vi "Pre Launch Init.vi"(11 "Series Actor in":refnum<class "Series Actor.lvclass">) -> (0 "error out":errorcluster, 3 "Series Actor out":refnum<class "Series Actor.lvclass">)   [LabVIEW 2023, in "HAL GOOP4.lvlib" / "Series Actor.lvlib" / "Series Actor.lvclass"]
doc: "(<B>Filename</B>: Actor Framework.lvlib:Actor.lvclass:Pre Launch Init.vi)\n\nDefines behavior that occurs after the Launch Nested Actor method is invoked but before the actor's Actor Core method begins running.\n\nBy default, this method does nothing. A descendant class may override it to define behavior."
uses:
  Series Actor.lvclass
  Series Actor.lvclass/Series Actor.ctl
  <vilib>/ActorFramework/Actor/Actor.lvclass
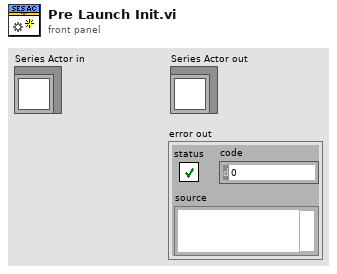
[diagram p1: front panel]
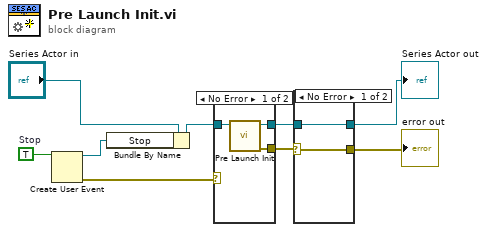
[diagram p0: block diagram]
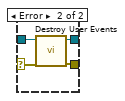
[diagram p2: hidden frame]
diagram:
  w8 = TRUE  # Stop
  n1 = Create User Event(user event datatype=w8) -> (user event=w1:refnum<user-event>, error out=w7:errorcluster)  [unwired: 1 in]
  n2 = Bundle By Name(cluster="Series Actor in", "Stop"=w1) -> (w2:refnum<class "Series Actor.lvclass">)
  n3 = case shown="No Error" w7 {
    selector: w7 -> [_ w14]
    tunnel: [w12 w14] -> w6
    tunnel: [w11 w13] -> w4
    tunnel: w2 -> [w10 w13]
    frame No Error {
      n4 = call-parent "Pre Launch Init.vi"("Actor in"=w10) -> ("error out"=w12:errorcluster, "Actor out"=w11:refnum<class "Series Actor.lvclass">)  [unwired: 9 in]
    }
    frame Error {
    }
  }
  n5 = case shown="No Error" w6 {
    selector: w6 -> [w16 w19]
    tunnel: [w16 w18] -> w5
    tunnel: w4 -> [w15 w20]
    tunnel: [w15 w17] -> w3
    frame No Error {
    }
    frame Error {
      n6 = call-dynamic "Destroy User Events.vi"("error in"=w19, "Series Actor in"=w20) -> ("error out"=w18:errorcluster, "Series Actor out"=w17:refnum<class "Series Actor.lvclass">)  [unwired: 8 in]
    }
  }
  "error out" <- w5
  "Series Actor out" <- w3
